vi "Directional Speed 1.0 Write Inputs.vi"(5 "Device inputs":dbl[](array[numeric]), 7 "Last Device inputs":dbl[](array[numeric]), 8 "error in (no error)":errorcluster, 9 "input reference in":T1, 10 "input in":T2, 11 "FIFO indexes.inputs":T3) -> (0 "error out":errorcluster, 1 "input reference out":T1, 2 "input out":T2)   [LabVIEW 2019, in "Engine Simulation Toolkit Engine.lvlib"]
uses:
  Engine Simulation Toolkit Engine.lvlib
  Shared/1.0 Directional Speed FIFO Idxs.ctl
  Directional Speed 1.0 Input Ref.ctl
  Shared/Engine Simulation Toolkit Shared.lvlib
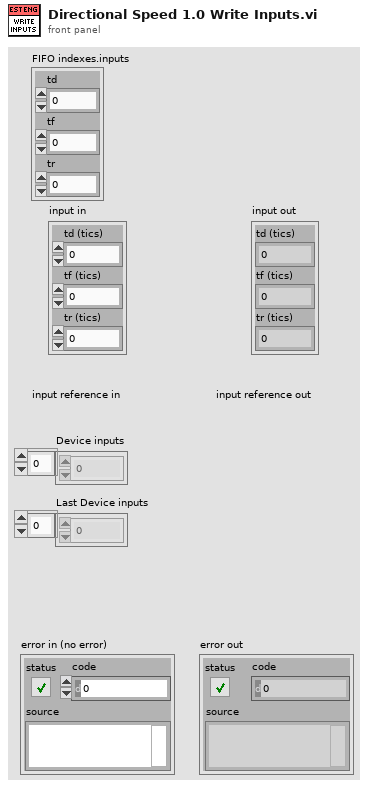
[diagram p1: front panel]
types:
  T1 = typedef "Engine Simulation Toolkit Engine.lvlib/Directional Speed 1.0 Input Ref.ctl" = refnum<k20>
  T2 = cluster{"td (tics)":u16, "tf (tics)":u16, "tr (tics)":u16}
  T3 = typedef "Engine Simulation Toolkit Shared.lvlib/1.0 Directional Speed FIFO Idxs.ctl" = cluster{"td":i32, "tf":i32, "tr":i32}
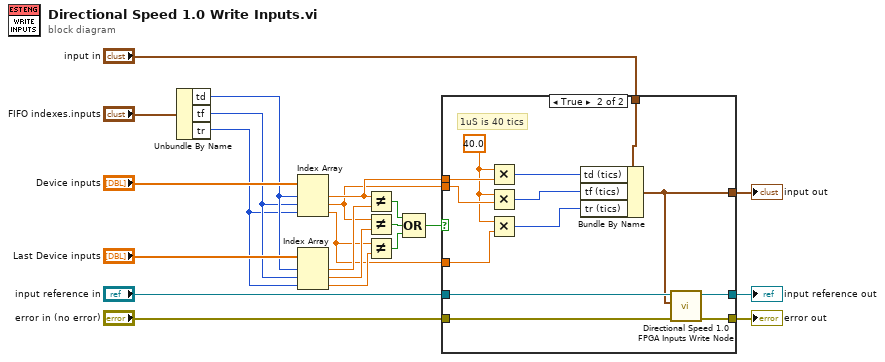
[diagram p0: block diagram]
diagram:
  n1 = Unbundle By Name("FIFO indexes.inputs") -> ("td"=w14:i32, "tf"=w2:i32, "tr"=w1:i32)
  n2 = Index Array(array="Device inputs", index #1=w14, index #2=w2, index #3=w1) -> (element #1=w11:dbl, element #2=w4:dbl, element #3=w3:dbl)
  n3 = Index Array(array="Last Device inputs", index #1=w14, index #2=w2, index #3=w1) -> (element #1=w12:dbl, element #2=w6:dbl, element #3=w5:dbl)
  n4 = Not Equal?(x=w11, y=w12) -> (x != y?=w10:bool)
  n5 = Not Equal?(x=w4, y=w6) -> (x != y?=w9:bool)
  n6 = Not Equal?(x=w3, y=w5) -> (x != y?=w8:bool)
  n7 = Compound Arithmetic op=OR(w10, w9, w8) -> (w7:bool)
  n8 = case shown="True" w7 {
    tunnel: "error in (no error)" -> [w23 w38]
    tunnel: "input reference in" -> [w24 w37]
    tunnel: [w23 w36] -> w20
    tunnel: [w24 w35] -> w19
    tunnel: "input in" -> [w25 w34]
    tunnel: [w25 w33] -> w13
    tunnel: w11 -> [_ w32]
    tunnel: w4 -> [_ w28]
    tunnel: w3 -> [_ w27]
    frame False {
    }
    frame True {
      w26 = 40.0
      # "1uS is 40 tics"
      n9 = Multiply(x=w26, y=w32) -> (x*y=w31:u16)
      n10 = Multiply(x=w26, y=w28) -> (x*y=w30:u16)
      n11 = Multiply(x=w26, y=w27) -> (x*y=w29:u16)
      n12 = Bundle By Name(cluster=w34, "td (tics)"=w31, "tf (tics)"=w30, "tr (tics)"=w29) -> (w33:T2)
      n13 = call "Directional Speed 1.0 FPGA Inputs Write Node.vi"("error in (no error)"=w38, "input"=w33, "Refnum in"=w37) -> ("error out"=w36:errorcluster, "Refnum out"=w35:T1)  [unwired: 7 in]
    }
  }
  "error out" <- w20
  "input out" <- w13
  "input reference out" <- w19
